vi "test Read Message (TCP) Shares Timeout.vi"(8 "error in (no error)":errorcluster, 11 "TestCase in":refnum<class "TCP API Tests.lvclass">) -> (0 "error out":errorcluster, 3 "TestCase out":refnum<class "TCP API Tests.lvclass">)   [LabVIEW 2013, in "TCP API Tests.lvclass"]
uses:
  TCP API Tests.lvclass
  vi.lib/NI/STM/TCP/TCP Read Options.ctl
  vi.lib/NI/STM/TCP/Write Meta Data (TCP Ref).vi
  vi.lib/NI/STM/TCP/Read Meta Data (TCP Ref).vi
  vi.lib/NI/STM/TCP/Write Meta Data (TCP Clst).vi
  vi.lib/NI/STM/TCP/Read Meta Data (TCP Clst).vi
  <vilib>/addons/_JKI Toolkits/VI Tester/TestCase.llb/TestCase.lvclass
  vi.lib/NI/STM/NI STM.lvlib
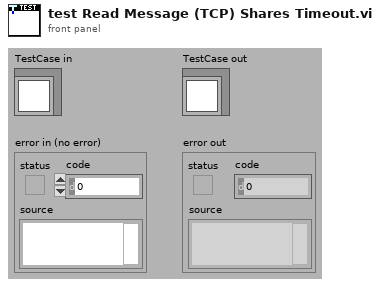
[diagram p1: front panel]
types:
  T1 = typedef "NI STM.lvlib/TCP Read Options.ctl" = cluster{"ignore timeout error":bool, "timeout ms (1000)":i32}
  T2 = typedef "NI STM.lvlib/TCP Connection Info.ctl" = cluster{"connection ID":refnum<k5>, "meta data":T3[]}
  T3 = typedef "NI STM.lvlib/MetaDataElement.ctl" = string
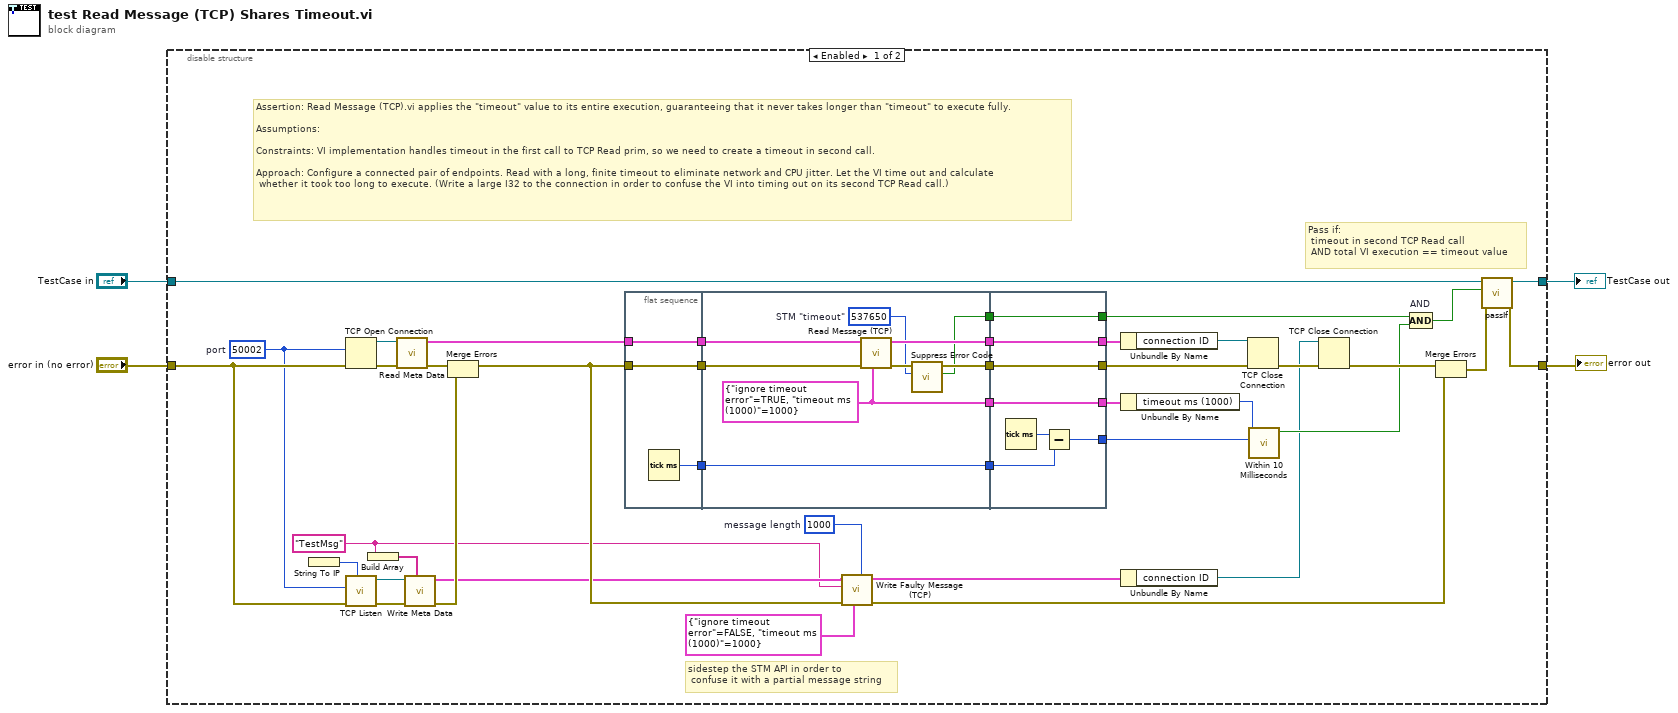
[diagram p0: block diagram]
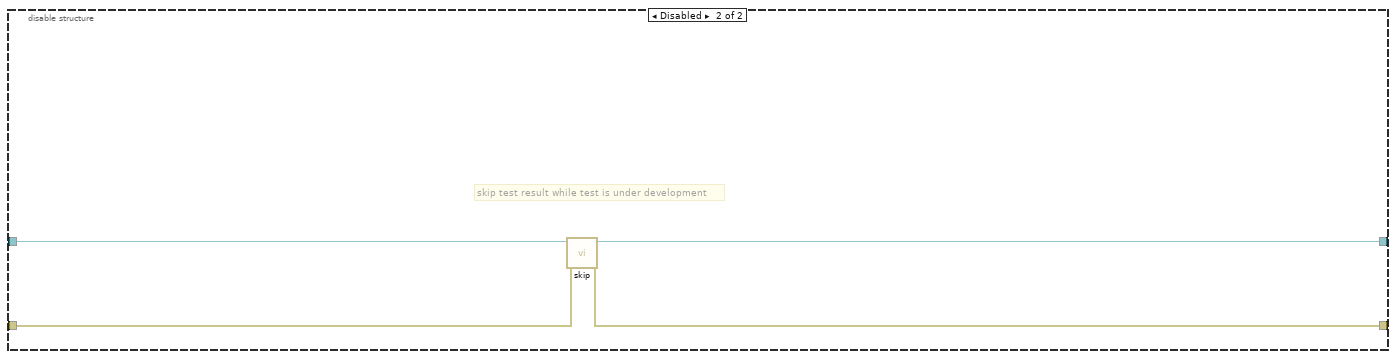
[diagram p2: hidden frame]
diagram:
  n1 = disable-structure shown="Enabled" {
    disable-tunnel: "TestCase in" -> [w46 w69]
    disable-tunnel: [w45 w67] -> w1
    disable-tunnel: [w44 w68] -> w3
    disable-tunnel: "error in (no error)" -> [w43 w66]
    frame Enabled {
      w5 = "TestMsg" ("Meta Element")
      w11 = i64 1000  # message length
      w42 = u16 50002  # port
      # "Pass if:\n timeout in second TCP Read call\n AND total VI execution == timeout value"
      # "sidestep the STM API in order to\n confuse it with a partial message string"
      # "Assertion: Read Message (TCP).vi applies the \"timeout\" value to its entire execution, guaranteeing that it never takes longer than \"timeout\" to execute fully.\n\nAssumptions: \n\nConstraints: VI implementation handles timeout in the first call to TCP Read prim, so we need to create a timeout in second call.\n\nApproach: Configure a connected pair of endpoints. Read with a long, finite timeout to eliminate network and CPU jitter. Let the VI time out and calculate\n whether it took too long to execute. (Write a large I32 to the connection in order to confuse the VI into timing out on its second TCP Read call.)"
      n2 = String To IP() -> (0:w41:u32)  [unwired: 1 in]
      n3 = TCP Open Connection(remote port or service name=w42, error in (no error)=w43) -> (connection ID=w40:refnum<k5>, error out=w24:errorcluster)  [unwired: 3 in]
      n4 = call <vilib>:"TCP Listen.vi"("net address"=w41, "error in (no error)"=w43, "port"=w42) -> ("error out"=w22:errorcluster, "connection ID"=w23:refnum<k5>)  [unwired: 4 in, 3 out]
      n5 = Build Array(w5) -> (w6:string[])
      n6 = call-poly "Read Meta Data.vi"("error in"=w24, "connection ID"=w40) -> ("error out"=w39:errorcluster, "connection info out"=w37:T2)  [unwired: 1 in, 7 out]
      n7 = call-poly "Write Meta Data.vi"("meta data"=w6, "error in"=w22, "connection ID"=w23) -> ("error out"=w21:errorcluster, "connection info out"=w9:T2)  [unwired: 2 in, 5 out]
      n8 = Merge Errors(w39, w21) -> (w12:errorcluster)
      n9 = flat-sequence {
        tunnel: w37 -> [w48]
        tunnel: w12 -> [w49]
        tunnel: [w49] -> w36
        tunnel: [w48] -> w35
        tunnel: [w47] -> w32
        tunnel: w36 -> [w58]
        tunnel: w35 -> [w56]
        tunnel: [w52] -> w34
        tunnel: [w55] -> w33
        tunnel: w32 -> [w55]
        tunnel: [w54] -> w31
        tunnel: [w53] -> w29
        tunnel: [w50] -> w19
        tunnel: [w65] -> w38
        tunnel: w34 -> [w65]
        tunnel: w33 -> [w63]
        tunnel: w31 -> [w62]
        tunnel: [w62] -> w30
        tunnel: [w61] -> w18
        tunnel: [w60] -> w28
        tunnel: w29 -> [w60]
        tunnel: [w59] -> w16
        tunnel: w19 -> [w59]
        frame #0 {
          n10 = Tick Count (ms)() -> (millisecond timer value=w47:u32)
        }
        frame #1 {
          w51 = 537650  # STM "timeout"
          w54 = T1 {"ignore timeout error"=TRUE, "timeout ms (1000)"=1000} ("options")
          n11 = call "Read Message (TCP).vi"("options"=w54, "error in"=w58, "connection info in"=w56) -> ("error out"=w57:errorcluster, "connection info out"=w53:T2)  [unwired: 3 in, 4 out]
          n12 = call "Suppress Error Code.vi"("Error Code"=w51, "Error In"=w57) -> ("Error Supressed?"=w50:bool, "Error Out"=w52:errorcluster)  [unwired: 4 in]
        }
        frame #2 {
          n13 = Tick Count (ms)() -> (millisecond timer value=w64:u32)
          n14 = Subtract(x=w64, y=w63) -> (x-y=w61:u32)
        }
      }
      n15 = call "Write Faulty Message (TCP).vi"("message length [bytes] (-1: calculate)"=w11, "options"=T1 {"ignore timeout error"=FALSE, "timeout ms (1000)"=1000}, "error in"=w12, "name (\"\")"=w5, "connection info in"=w9) -> ("error out"=w13:errorcluster, "connection info out"=w8:T2)  [unwired: 5 in]
      n16 = Unbundle By Name(w28) -> ("connection ID"=w27:refnum<k5>)
      n17 = Unbundle By Name(w30) -> ("timeout ms (1000)"=w17:i32)
      n18 = Unbundle By Name(w8) -> ("connection ID"=w7:refnum<k5>)
      n19 = TCP Close Connection(connection ID=w27, error in (no error)=w38) -> (error out=w26:errorcluster)  [unwired: 1 in, 1 out]
      n20 = call "Within 10 Milliseconds.vi"("milliseconds 2"=w18, "milliseconds 1"=w17) -> ("within 10 ms"=w15:bool)  [unwired: 9 in]
      n21 = TCP Close Connection(connection ID=w7, error in (no error)=w26) -> (error out=w25:errorcluster)  [unwired: 1 in, 1 out]
      n22 = Compound Arithmetic op=AND "AND"(w16, w15) -> (w14:bool)
      n23 = Merge Errors(w25, w13) -> (w20:errorcluster)
      n24 = call-dynamic "passIf.vi"("error in (no error)"=w20, "pass"=w14, "TestCase in"=w46) -> ("error out"=w44:errorcluster, "TestCase out"=w45:refnum<class "TCP API Tests.lvclass">)  [unwired: 7 in]
    }
    frame Disabled {
      # "skip test result while test is under development"
      n25 = call <vilib>:"skip.vi"("error in (no error)"=w66, "TestCase in"=w69) -> ("error out"=w68:errorcluster, "TestCase out"=w67:refnum<class "TCP API Tests.lvclass">)  [unwired: 8 in]
    }
  }
  "error out" <- w3
  "TestCase out" <- w1
